vi "Initialize Measurement Actor Core.vi"(5 "Title Ref":refnum<vi>, 7 "Wvfm Graph Ref":refnum<vi>, 8 "error in (no error)":errorcluster, 10 "Iteration":refnum<vi>, 11 "Measurement in":refnum<class "Measurement.lvclass">) -> (0 "error out":errorcluster, 1 "event out":refnum<user-event>, 2 "notifier out":refnum<notifier>, 3 "Measurement out":refnum<class "Measurement.lvclass">)   [LabVIEW 2026, in "Measurement Actor.lvlib" / "Measurement.lvclass"]
uses:
  Measurement.lvclass
  C:/Program Files/National Instruments/LabVIEW 2026/vi.lib/ActorFramework/Actor/Actor.lvclass
  Measurement.lvclass/Measurement.ctl
  <vilib>/ActorFramework/Actor/Actor.lvclass/Actor.ctl
  <vilib>/ActorFramework/Message Enqueuer/Message Enqueuer.lvclass/Message Enqueuer.ctl
  <vilib>/ActorFramework/Message Enqueuer/Enqueue.vi
  <vilib>/ActorFramework/Message Enqueuer/Init from Existing Queue.vi
  Messages/Configure Msg/Configure Msg.lvclass
  C:/Program Files/National Instruments/LabVIEW 2026/vi.lib/ActorFramework/Message/Message.lvclass
  Accessors/Write Iteration.vi
  <vilib>/ActorFramework/Message Priority Queue/Priority Enqueue.vi
  <vilib>/ActorFramework/Message Enqueuer/Message Enqueuer.lvclass
  <vilib>/ActorFramework/Actor/Actor.lvclass
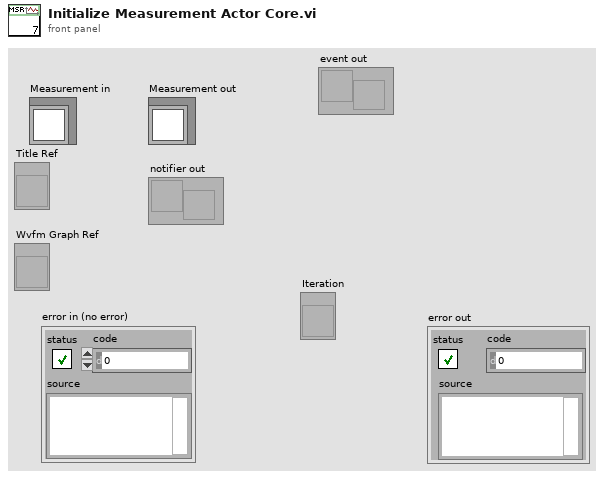
[diagram p1: front panel]
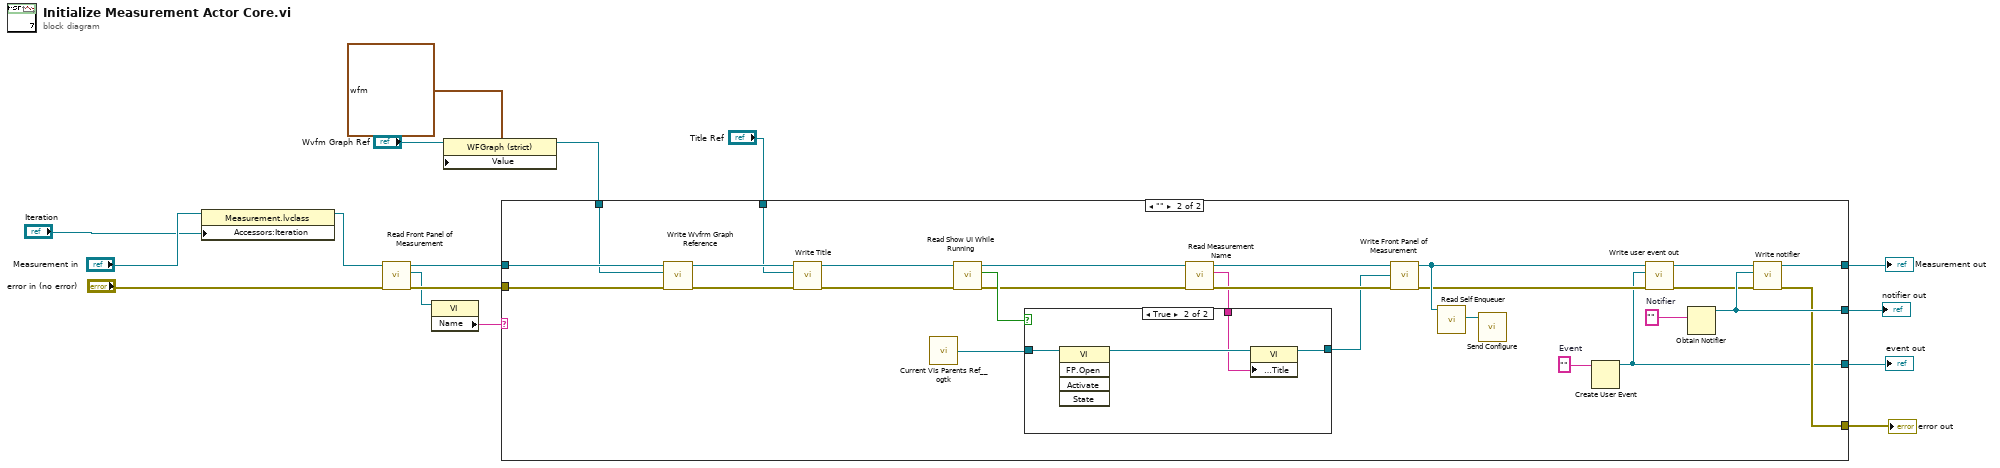
[diagram p0: block diagram]
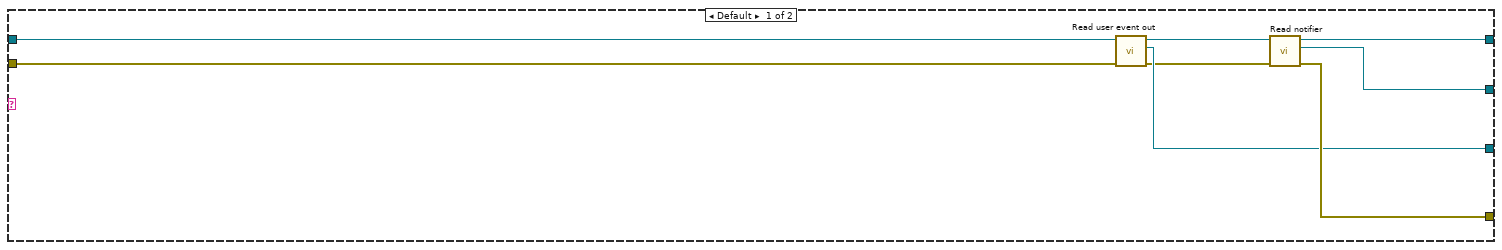
[diagram p2: hidden frame]
diagram:
  n1 = property class="Measurement.lvclass"(reference="Measurement in", "Accessors:Iteration"="Iteration") -> (reference out=w1:refnum<class "Measurement.lvclass">)  [unwired: 1 in, 1 out]
  n2 = call "Read Front Panel of Measurement.vi"("error in (no error)"="error in (no error)", "Measurement in"=w1) -> ("error out"=w14:errorcluster, "Front Panel of Measurement"=w13:refnum<vi>, "Measurement out"=w15:refnum<class "Measurement.lvclass">)  [unwired: 7 in]
  n3 = property class="VI"(reference=w13) -> ("Name"=w12:string)  [unwired: 1 in, 2 out]
  n4 = property class="WFGraph (strict)"(reference="Wvfm Graph Ref", "Value"=waveform(dbl) {"t0"=timestamp(0 s since 1904-01-01), "dt"=1.0, "Y"=[]}) -> (reference out=w5:refnum<vi>)  [unwired: 1 in, 1 out]
  n5 = case shown="\"\"" w12 {
    tunnel: [w24 w50] -> w10
    tunnel: w15 -> [w21 w32]
    tunnel: w14 -> [w18 w31]
    tunnel: [w23 w49] -> w11
    tunnel: [w22 w48] -> w9
    tunnel: [w19 w33] -> w8
    tunnel: "Title Ref" -> [_ w26]
    tunnel: w5 -> [_ w25]
    frame Default {
      n6 = call "Read user event out.vi"("error in (no error)"=w18, "Measurement in"=w21) -> ("error out"=w17:errorcluster, "user event out"=w19:refnum<user-event>, "Measurement out"=w20:refnum<class "Measurement.lvclass">)  [unwired: 7 in]
      n7 = call "Read notifier.vi"("error in (no error)"=w17, "Measurement in"=w20) -> ("error out"=w22:errorcluster, "notifier"=w23:refnum<notifier>, "Measurement out"=w24:refnum<class "Measurement.lvclass">)  [unwired: 7 in]
    }
    frame "" {
      w38 = ""  # Event
      w51 = ""  # Notifier
      n8 = call "Write Wvfrm Graph Reference.vi"("error in (no error)"=w31, "General Measurement UI"=w25, "Measurement in"=w32) -> ("error out"=w30:errorcluster, "Measurement out"=w29:refnum<class "Measurement.lvclass">)  [unwired: 7 in]
      n9 = call "Write Title.vi"("error in (no error)"=w30, "Title"=w26, "Measurement in"=w29) -> ("error out"=w28:errorcluster, "Measurement out"=w27:refnum<class "Measurement.lvclass">)  [unwired: 7 in]
      n10 = call <userlib>:"Current VIs Parents Ref__ogtk.vi"() -> ("Calling VI's Reference"=w46:refnum<vi>)  [unwired: 2 in]
      n11 = call "Read Show UI While Running.vi"("error in (no error)"=w28, "Measurement in"=w27) -> ("error out"=w43:errorcluster, "Show UI While Running"=w45:bool, "Measurement out"=w44:refnum<class "Measurement.lvclass">)  [unwired: 7 in]
      n12 = call "Read Measurement Name.vi"("error in (no error)"=w43, "Measurement in"=w44) -> ("error out"=w42:errorcluster, "Measurement Name"=w39:string, "Measurement out"=w41:refnum<class "Measurement.lvclass">)  [unwired: 7 in]
      n13 = case shown="True" w45 {
        tunnel: w46 -> [w52 w56]
        tunnel: [w52 w54] -> w40
        tunnel: w39 -> [_ w53]
        frame False {
        }
        frame True {
          n14 = invoke class="VI" method="FP.Open"(reference=w56) -> (reference out=w55:refnum<vi>)  [unwired: 4 in, 4 out]
          n15 = property class="VI"(reference=w55, "Front Panel.Title"=w53) -> (reference out=w54:refnum<vi>)  [unwired: 1 in, 1 out]
        }
      }
      n16 = call "Write Front Panel of Measurement.vi"("error in (no error)"=w42, "Front Panel of Measurement"=w40, "Measurement in"=w41) -> ("error out"=w35:errorcluster, "Measurement out"=w37:refnum<class "Measurement.lvclass">)  [unwired: 7 in]
      n17 = call <vilib>:"Read Self Enqueuer.vi"("Actor"=w37) -> ("Self Enqueuer"=w47:refnum<class "Message Enqueuer.lvclass">)  [unwired: 10 in]
      n18 = call "Send Configure.vi"("Message Enqueuer in"=w47) -> ()  [unwired: 9 in, 2 out]
      n19 = Create User Event(user event datatype=w38) -> (user event=w33:refnum<user-event>)  [unwired: 1 in, 1 out]
      n20 = call "Write user event out.vi"("error in (no error)"=w35, "user event out"=w33, "Measurement in"=w37) -> ("error out"=w34:errorcluster, "Measurement out"=w36:refnum<class "Measurement.lvclass">)  [unwired: 7 in]
      n21 = Obtain Notifier(notification data type=w51) -> (notifier out=w49:refnum<notifier>)  [unwired: 3 in, 2 out]
      n22 = call "Write notifier.vi"("error in (no error)"=w34, "notifier"=w49, "Measurement in"=w36) -> ("error out"=w48:errorcluster, "Measurement out"=w50:refnum<class "Measurement.lvclass">)  [unwired: 7 in]
    }
  }
  "Measurement out" <- w10
  "error out" <- w9
  "notifier out" <- w11
  "event out" <- w8
